vi "Write Or Not.vi"(1 "Time":timestamp, 3 "data in":variant) -> (0 "Write?":bool)   [LabVIEW 2019, in "Logger.PGSQL.lvclass"]
uses:
  Logger.PGSQL.lvclass
  <userlib>/LevyLab/LV-Data/LV-Data.PG/LV-Data.PGSQL.lvclass
  <vilib>/Utility/Data Type/NI_Data Type.lvlib
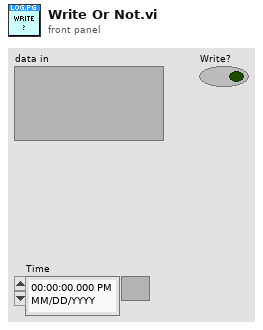
[diagram p1: front panel]
types:
  T1 = typedef "NI_Data Type.lvlib/Data Type.ctl" = enum8{"Invalid Type", "Void", "I8", "I16", "I32", "I64", "U8", "U16", "U32", "U64", "Single Float", "Double Float", "Extended Float", "Single Complex", "Double Complex", "Extended Complex", "Enum U8", "Enum U16", "Enum U32", "Enum U64", "Single Float With Unit", "Double Float With Unit", "Extended Float With Unit", "Single Complex with Unit", "Double Complex with Unit", "Extended Complex with Unit", "Boolean", "String", "Path", "Picture", "Tag", "Array", "Cluster", "Variant", "LV Variant", "Waveform", "Timestamp", "Digital Waveform", "Digital Data", "ExpressData", "Refnum", "External Data", "VI", "Poly VI", "LabVIEW Class Instance", "Fixed Point", "Set Collection", "Map Collection"}
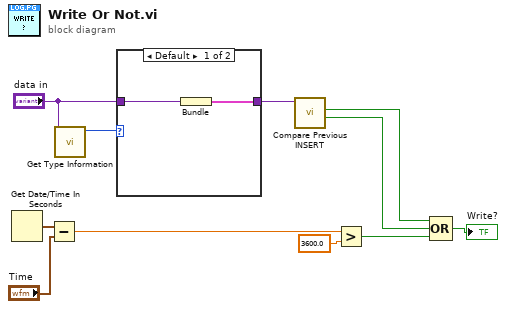
[diagram p0: block diagram]
diagram:
  n1 = Get Date/Time In Seconds() -> (seconds since 1Jan1904=w6:timestamp)
  n2 = Subtract(x=w6, y="Time") -> (x-y=w8:dbl)
  n3 = call <vilib>:"Get Type Information.vi"("variant"="data in") -> ("type"=w3:T1)  [unwired: 6 in, 4 out]
  n4 = case shown="Default" w3 {
    tunnel: "data in" -> [w13 w14]
    tunnel: [w12 w14] -> w1
    frame Default {
      n5 = Bundle("data in"=w13) -> (w12:cluster{"data in":variant})  [unwired: 1 in]
    }
    frame "Array", "Cluster" {
    }
  }
  n6 = call <userlib>:"Compare Previous INSERT.vi"("Data"=w1) -> ("Some Different"=w5:bool, "All Different"=w4:bool)  [unwired: 7 in, 2 out]
  n7 = Greater?(x=w8, y=3600.0) -> (0:w10:bool)
  n8 = Compound Arithmetic op=OR(w4, w5, w10) -> (→"Write?":bool)
